vi "Example Callback.vi"() -> ()   [LabVIEW 2010]
uses:
  C:/tf/play/labview/Tinkerforge.dll
  Tinkerforge.dll
panel:
  out "station  temperature (°C)":sgl format="%#_13g"
  out "station identifier":u8
  out "station humidity (%RH)":u8
  out "station wind speed (m/s)":sgl format="%.2f"
  out "station gust speed (m/s)":sgl format="%.2f"
  out "station rain":sgl format="%.2f"
  out "station wind direction":u8
  out "station battery low":bool
  out "sensor humidity (%RH)":u8
  out "sensor identifier":u8
  in  "stop":bool
  out "sensor temperature (°C)":sgl format="%#_13g"
  in  "uid":string="Fax"
  in  "port":i32=4223
  in  "host":string="localhost"
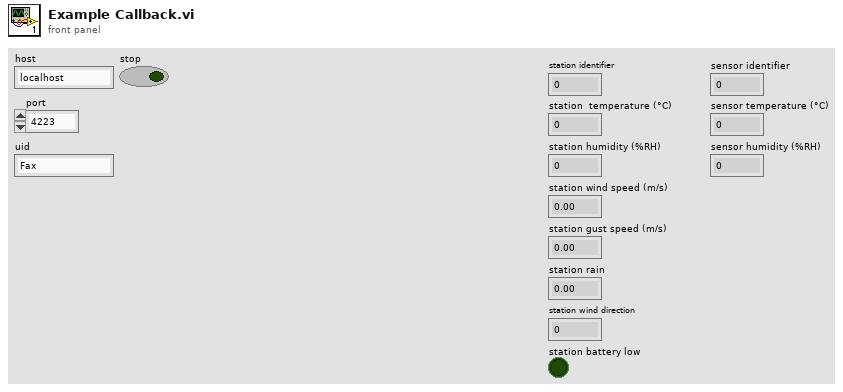
[diagram p1: front panel]
types:
  T1 = cluster{"identifier":u8, "temperature":i16, "humidity":u8, "windSpeed":i64, "gustSpeed":i64, "rain":i64, "windDirection":u8, "batteryLow":bool}
  T2 = cluster{"identifier":u8, "temperature":i16, "humidity":u8}
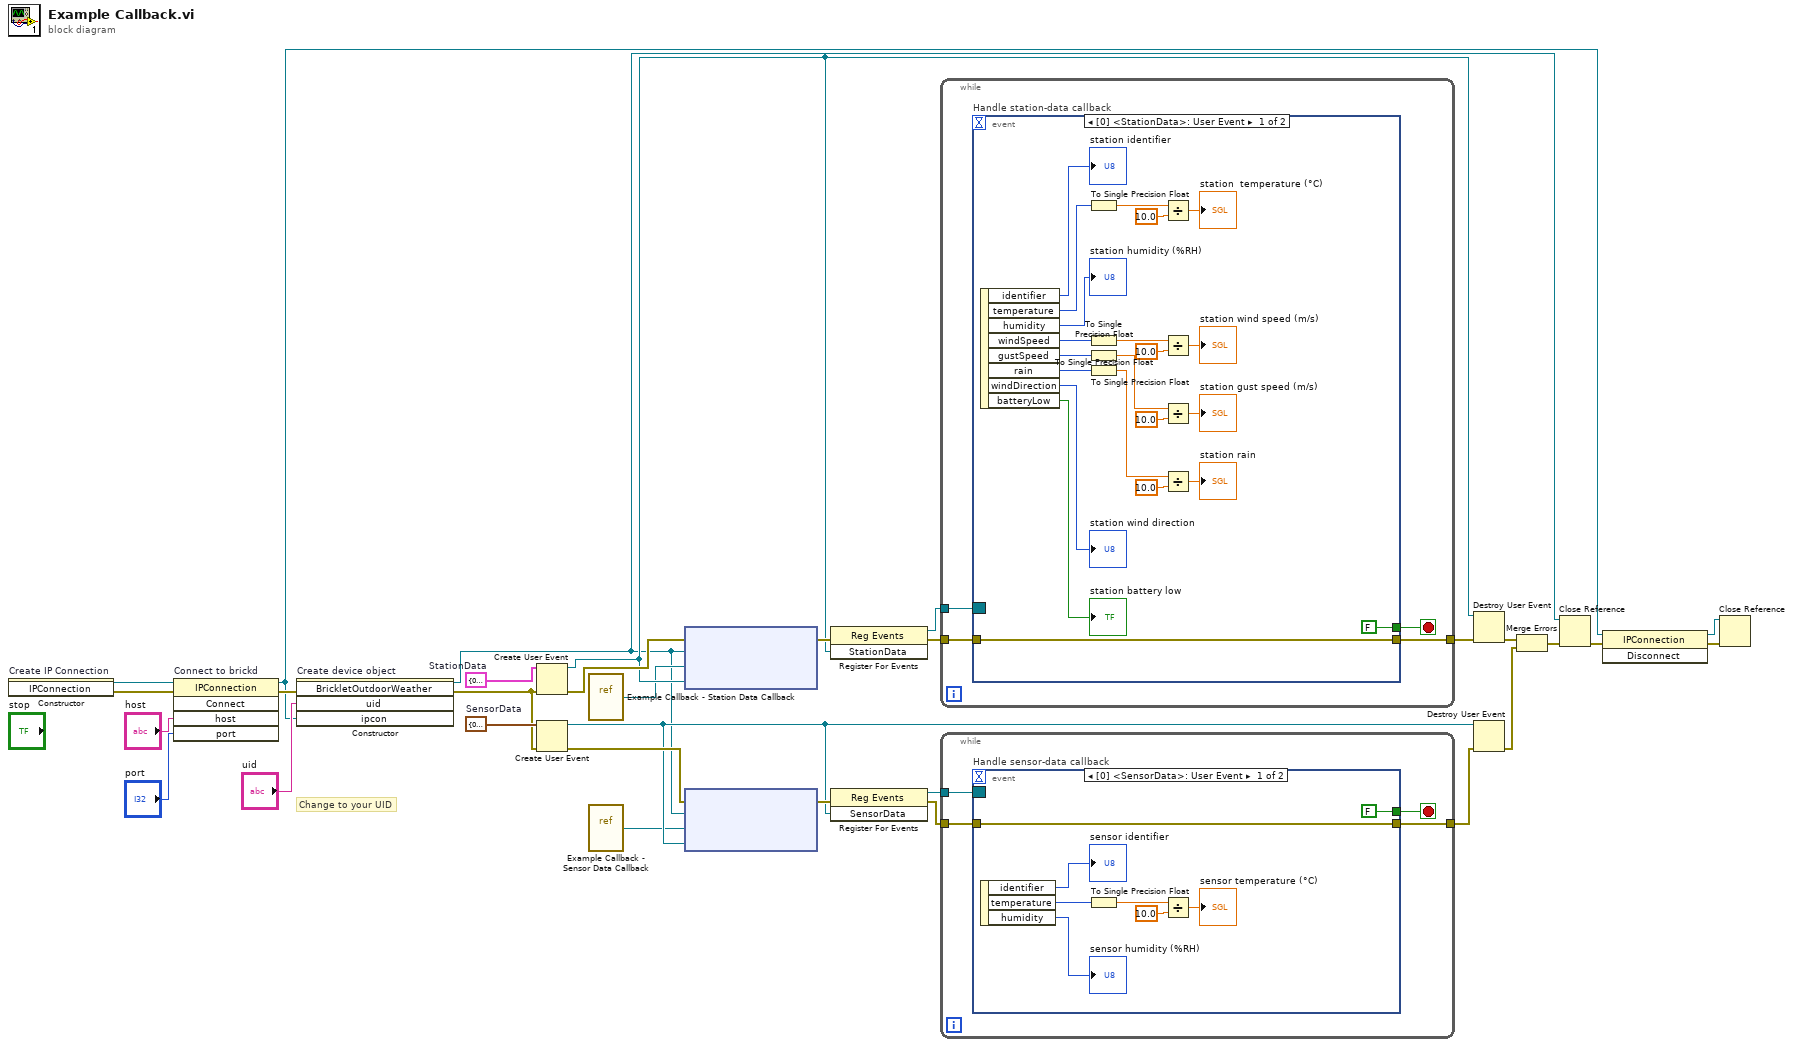
[diagram p0: block diagram]
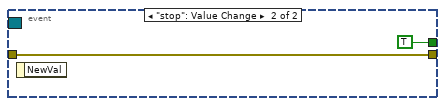
[diagram p2: hidden frame]
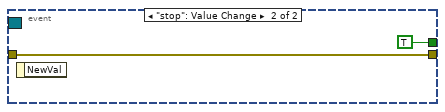
[diagram p3: hidden frame]
diagram:
  w10 = T1 {"identifier"=0, "temperature"=0, "humidity"=0, "windSpeed"=0, "gustSpeed"=0, "rain"=0, "windDirection"=0, "batteryLow"=TRUE}  # StationData
  w17 = T2 {"identifier"=0, "temperature"=0, "humidity"=0}  # SensorData
  # "Change to your UID"
  n1 = constructor on="Create IP Connection" class="IPConnection"() -> (reference out=w31:refnum<k24>, error out=w16:errorcluster)  [unwired: 3 in, 1 out]
  n2 = invoke on="Connect to brickd" class="IPConnection" method="Connect"(reference=w31, error in=w16, "host"="host", "port"="port") -> (reference out=w24:refnum<k24>, error out=w27:errorcluster)  [unwired: 1 in, 3 out]
  n3 = constructor on="Create device object" class="BrickletOutdoorWeather"(error in=w27, "uid"="uid", "ipcon"=w24) -> (reference out=w2:refnum<k24>, error out=w1:errorcluster)  [unwired: 2 in, 3 out]
  n4 = Create User Event(user event datatype=w10, error in=w1) -> (user event=w11:refnum<user-event>, error out=w15:errorcluster)
  n5 = Create User Event(user event datatype=w17, error in=w1) -> (user event=w18:refnum<user-event>, error out=w22:errorcluster)
  n6 = vi-ref "Example Callback - Station Data Callback.vi"() -> ("vi reference"=w9:refnum<vi>)
  n7 = vi-ref "Example Callback - Sensor Data Callback.vi"() -> ("vi reference"=w3:refnum<vi>)
  n8 = node ("Register Event Callback")(w15, w2, w9, w11) -> (w14:errorcluster)  [unwired: 1 in, 1 out]
  n9 = node ("Register Event Callback")(w22, w2, w3, w18) -> (w21:errorcluster)  [unwired: 1 in, 1 out]
  n10 = register-events(error in=w14, w11) -> (reference out=w13:refnum<event-registration>, error out=w12:errorcluster)  [unwired: 1 in]
  n11 = register-events(error in=w21, w18) -> (reference out=w20:refnum<event-registration>, error out=w19:errorcluster)  [unwired: 1 in]
  n12 = while {
    tunnel: w13 -> [w35]
    tunnel: [w34] -> w7
    tunnel: w12 -> [w33]
    stop <- w32 stop-if-true
    n13 = event "Handle station-data callback" shown="[0] <StationData>: User Event" {
      selector: w35 -> [_ _]
      dyn-events: _ -> [_ _]
      timeout: _ -> [_ _]
      tunnel: [w55 w58] -> w34
      tunnel: w33 -> [w55 w58]
      tunnel: [FALSE TRUE] -> w32
      event User Event {
        n14 = event-data() -> ("identifier"=→"station identifier":u8, "temperature"=w52:i16, "humidity"=→"station humidity (%RH)":u8, "windSpeed"=w47:i64, "gustSpeed"=w42:i64, "rain"=w40:i64, "windDirection"=→"station wind direction":u8, "batteryLow"=→"station battery low":bool)  [unwired: 1 in]
        n15 = To Single Precision Float(number=w52) -> (single precision float=w56:sgl)
        n16 = To Single Precision Float(number=w47) -> (single precision float=w48:sgl)
        n17 = To Single Precision Float(number=w42) -> (single precision float=w44:sgl)
        n18 = To Single Precision Float(number=w40) -> (single precision float=w41:sgl)
        n19 = Divide(x=w56, y=sgl 10.0) -> (x/y=→"station  temperature (°C)":sgl)
        n20 = Divide(x=w48, y=sgl 10.0) -> (x/y=→"station wind speed (m/s)":sgl)
        n21 = Divide(x=w44, y=sgl 10.0) -> (x/y=→"station gust speed (m/s)":sgl)
        n22 = Divide(x=w41, y=sgl 10.0) -> (x/y=→"station rain":sgl)
      }
      event "stop": Value Change {
        n23 = event-data() -> ()  [unwired: 1 in, 1 out]
      }
    }
  }
  n24 = while {
    tunnel: w20 -> [w63]
    tunnel: [w62] -> w8
    tunnel: w19 -> [w61]
    stop <- w60 stop-if-true
    n25 = event "Handle sensor-data callback" shown="[0] <SensorData>: User Event" {
      selector: w63 -> [_ _]
      dyn-events: _ -> [_ _]
      timeout: _ -> [_ _]
      tunnel: [w69 w72] -> w62
      tunnel: w61 -> [w69 w72]
      tunnel: [FALSE TRUE] -> w60
      event User Event {
        n26 = event-data() -> ("identifier"=→"sensor identifier":u8, "temperature"=w66:i16, "humidity"=→"sensor humidity (%RH)":u8)  [unwired: 1 in]
        n27 = To Single Precision Float(number=w66) -> (single precision float=w70:sgl)
        n28 = Divide(x=w70, y=sgl 10.0) -> (x/y=→"sensor temperature (°C)":sgl)
      }
      event "stop": Value Change {
        n29 = event-data() -> ()  [unwired: 1 in, 1 out]
      }
    }
  }
  n30 = Destroy User Event(user event=w11, error in=w7) -> (error out=w6:errorcluster)
  n31 = Destroy User Event(user event=w18, error in=w8) -> (error out=w5:errorcluster)
  n32 = Merge Errors(w6, w5) -> (w4:errorcluster)
  n33 = Close Reference(reference=w2, error in (no error)=w4) -> (error out=w26:errorcluster)
  n34 = invoke class="IPConnection" method="Disconnect"(reference=w24, error in=w26) -> (reference out=w23:refnum<k24>, error out=w25:errorcluster)  [unwired: 1 in, 1 out]
  n35 = Close Reference(reference=w23, error in (no error)=w25) -> ()  [unwired: 1 out]
